vi "EnterComms.vi"(8 "error in (no error)":errorcluster) -> (0 "error out":errorcluster, 2 "Cancelled?":bool, 3 "Comunicaciones":T1={"Flujo_1"="COM4", "Brk1"=TRUE, "Flujo_2"="COM6", "Brk2"=TRUE, "Flujo_3"="COM8", "Brk3"=FALSE, "Flujo_4"="COM10", "Brk4"=FALSE, "Eurothe"="COM5", "Eurot"=FALSE, "Balanza"="COM7", "Bal"=FALSE, "eValPos"="COM9", "eVal"=FALSE, "flowbus"="COM29", "fb"=FALSE})   [LabVIEW 2013]
doc: "Use this template to create a dialog box. This template polls the state of the buttons on the front panel and does not use events. Use the Dialog Using Events template (not available in Base package) to create a dialog box with event handling."
uses:
  Controles/P2018 Com Control.ctl
panel:
  in  "Bal":bool=TRUE
  in  "Eurot":bool=TRUE
  in  "eVal":bool=TRUE
  in  "fw":bool=TRUE
  in  "Balanza":refnum<visa-resource-name>="COM9" caption="C1.6"
  in  "EV&Posicion":refnum<visa-resource-name>="COM10" caption="C1.7"
  in  "Eurotherm":refnum<visa-resource-name>="COM8" caption="C1.5"
  in  "Flowbus":refnum<visa-resource-name>="COM3" caption="C1.8"
  out "Enable":bool=TRUE
  out "Disable":bool
  in  "Brk3":bool=TRUE
  in  "Brk1":bool=TRUE
  in  "Brk2":bool=TRUE
  in  "Brk4":bool=TRUE
  in  "Flujo_3":refnum<visa-resource-name>="COM6" caption="C1.3"
  in  "Flujo_2":refnum<visa-resource-name>="COM5" caption="C1.2"
  in  "Flujo_1":refnum<visa-resource-name>="COM4" caption="C1.1"
  in  "Flujo_4":refnum<visa-resource-name>="COM7" caption="C1.4"
  in  "Cancel":bool
  in  "OK":bool
  # "Comunicaciones"
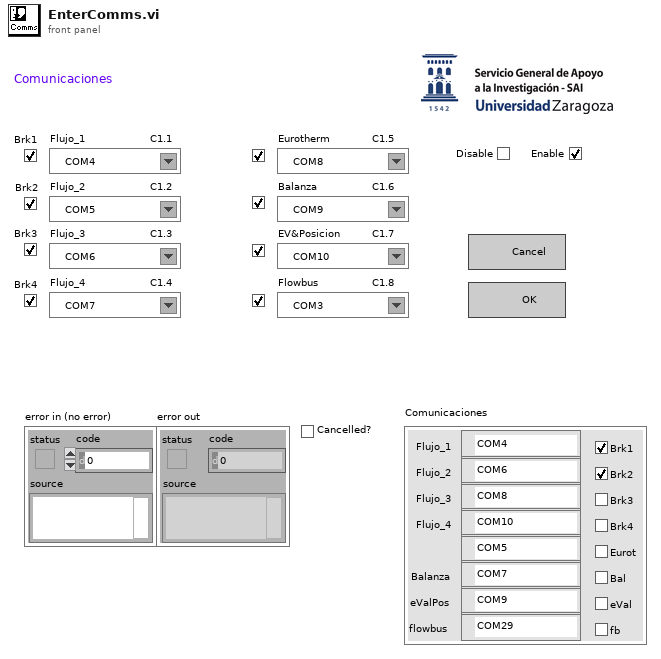
[diagram p1: front panel]
types:
  T1 = typedef "P2018 Com Control.ctl" = cluster{"Flujo_1":refnum<visa-resource-name>, "Brk1":bool, "Flujo_2":refnum<visa-resource-name>, "Brk2":bool, "Flujo_3":refnum<visa-resource-name>, "Brk3":bool, "Flujo_4":refnum<visa-resource-name>, "Brk4":bool, "Eurothe":refnum<visa-resource-name>, "Eurot":bool, "Balanza":refnum<visa-resource-name>, "Bal":bool, "eValPos":refnum<visa-resource-name>, "eVal":bool, "flowbus":refnum<visa-resource-name>, "fb":bool}
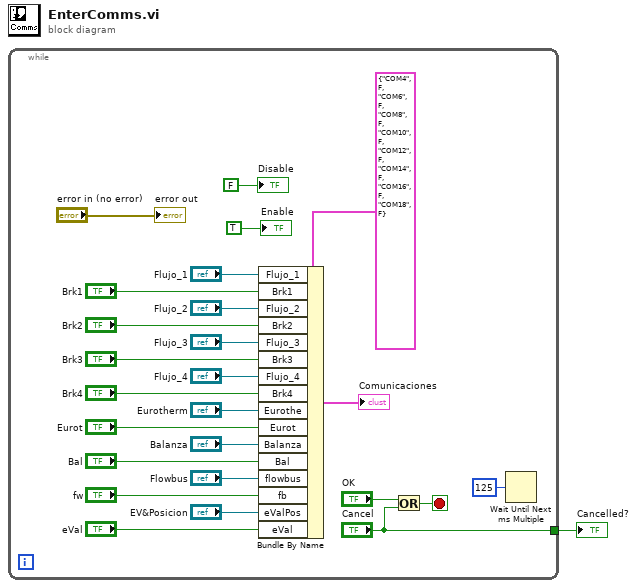
[diagram p0: block diagram]
diagram:
  n1 = while {
    tunnel: ["Cancel"] -> w1
    stop <- w25 stop-if-true
    n2 = Bundle By Name(cluster=T1 {"Flujo_1"="COM4", "Brk1"=FALSE, "Flujo_2"="COM6", "Brk2"=FALSE, "Flujo_3"="COM8", "Brk3"=FALSE, "Flujo_4"="COM10", "Brk4"=FALSE, "Eurothe"="COM12", "Eurot"=FALSE, "Balanza"="COM14", "Bal"=FALSE, "eValPos"="COM16", "eVal"=FALSE, "flowbus"="COM18", "fb"=FALSE} ("Comunicaciones"), "Flujo_1"="Flujo_1", "Brk1"="Brk1", "Flujo_2"="Flujo_2", "Brk2"="Brk2", "Flujo_3"="Flujo_3", "Brk3"="Brk3", "Flujo_4"="Flujo_4", "Brk4"="Brk4", "Eurothe"="Eurotherm", "Eurot"="Eurot", "Balanza"="Balanza", "Bal"="Bal", "flowbus"="Flowbus", "fb"="fw", "eValPos"="EV&Posicion", "eVal"="eVal") -> (→"Comunicaciones":T1)
    n3 = Or(x="OK", y="Cancel") -> (x .or. y?=w25:bool)
    n4 = Wait Until Next ms Multiple(millisecond multiple=u32 125) -> ()  [unwired: 1 out]
    "error out" <- "error in (no error)"
    "Disable" <- FALSE ("No usado")
    "Enable" <- TRUE ("Si usado")
  }
  "Cancelled?" <- w1
